vi "GUI.vi"(11 "Trace Queue":refnum<queue>) -> ()   [LabVIEW 2018]
uses:
  <vilib>/Utility/miscctls.llb/LVRowAndColumnUnsignedTypeDef.ctl
panel:
  out "Trace":string[][](table)
  in  "Size":i32=1000 format="%d lines"
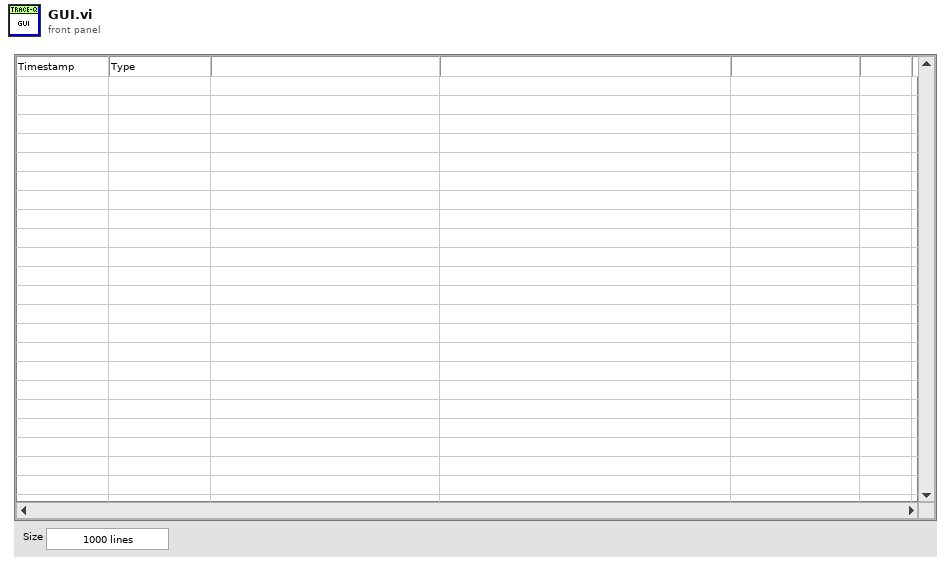
[diagram p1: front panel]
types:
  T1 = typedef "LVRowAndColumnUnsignedTypeDef.ctl" = cluster{"Row":u32, "Column":u32}
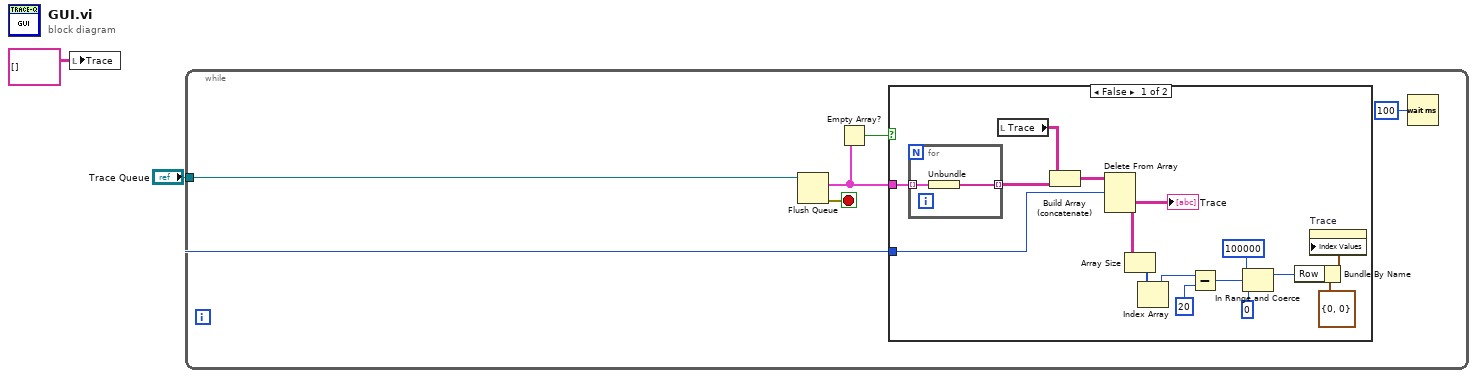
[diagram p0: block diagram]
diagram:
  n1 = local write "Trace"(string[][] [] ("Trace")) -> ()
  n2 = while {
    tunnel: "Trace Queue" -> [w3]
    stop <- w8 stop-if-true
    n3 = Flush Queue(queue=w3) -> (remaining elements=w4:cluster{string[]}[], error out=w8:errorcluster)  [unwired: 1 in, 1 out]
    n4 = Empty Array?(array=w4) -> (empty?=w5:bool)
    n5 = case shown="False" w5 {
      tunnel: "Size" -> [w20 _]
      tunnel: w4 -> [w19 _]
      frame False {
        n6 = for {
          tunnel: w19 -> [w25] mode=indexing
          tunnel: [w24] -> w22 mode=indexing
          n7 = Unbundle(w25) -> (w24:string[])
        }
        n8 = local read "Trace"() -> (w23:string[][])
        n9 = Build Array (concatenate)(w23, w22) -> (w21:string[][])
        n10 = Delete From Array(array=w21, length=w20) -> (deleted portion=w16:string[][])  [unwired: 2 in, 1 out]
        "Trace" <- w16
        n11 = Array Size(array=w16) -> (size(s)=w15:i32[])
        n12 = Index Array(array=w15) -> (element=w14:i32)  [unwired: 1 in]
        n13 = Subtract(x=w14, y=20) -> (x-y=w10:i32)
        n14 = In Range and Coerce(upper limit=100000, x=w10, lower limit=0) -> (coerced(x)=w13:i32)  [unwired: 1 out]
        n15 = Bundle By Name(cluster=T1 {"Row"=0, "Column"=0} ("Index Values"), "Row"=w13) -> (w17:T1)
        n16 = property on="Trace" class="Tbl (strict)"("Index Values"=w17) -> ()  [unwired: 2 in, 2 out]
      }
      frame True {
      }
    }
    n17 = Wait (ms)(milliseconds to wait=u32 100) -> ()  [unwired: 1 out]
  }
